vi "Test.vi"() -> ()   [LabVIEW 2013, in "Standard Editor.lvlib" / "splash screen.lvlib"]
uses:
  splash screen.lvlib
  notifier data.ctl
panel:
  out "error out":errorcluster
  in  "error in":errorcluster
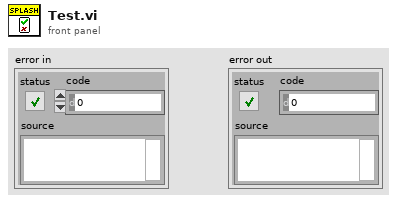
[diagram p1: front panel]
types:
  T1 = typedef "Standard Editor.lvlib/splash screen.lvlib/splash screen.ctl" = cluster{"reference":refnum<vi>, "update notifier":refnum<notifier>, "Initialized":bool}
  T2 = typedef "Standard Editor.lvlib/splash screen.lvlib/notifier data.ctl" = cluster{"Text":string, "percent":dbl}
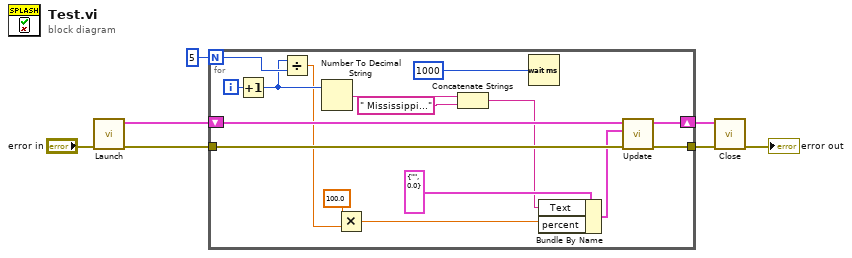
[diagram p0: block diagram]
diagram:
  n1 = call "Launch.vi"("error in"="error in") -> ("error out"=w5:errorcluster, "SplashScreen"=w6:T1)  [unwired: 9 in]
  n2 = for {
    N: 5 -> [w20]
    tunnel: w5 -> [w22]
    tunnel: [w15] -> w2
    shift-right: [w16] -> w3
    shift-left: w6 -> [w23]
    i -> [w21]
    n3 = Increment(x=w21) -> (x+1=w19:i32)
    n4 = Divide(x=w19, y=w20) -> (x/y=w10:dbl)
    n5 = Number To Decimal String(number=w19) -> (decimal integer string=w12:string)  [unwired: 1 in]
    n6 = Multiply(x=100.0, y=w10) -> (x*y=w8:dbl)
    n7 = Concatenate Strings(w12, " Mississippi...") -> (w11:string)
    n8 = Wait (ms)(milliseconds to wait=u32 1000) -> ()  [unwired: 1 out]
    n9 = Bundle By Name(cluster=T2 {"Text"="", "percent"=0.0} ("Update"), "Text"=w11, "percent"=w8) -> (w17:T2)
    n10 = call "Update.vi"("error in"=w22, "Update"=w17, "SplashScreen in"=w23) -> ("error out"=w15:errorcluster, "SplashScreen out"=w16:T1)  [unwired: 7 in]
  }
  n11 = call "Close.vi"("error in"=w2, "SplashScreen"=w3) -> ("error out"=→"error out":errorcluster)  [unwired: 8 in, 1 out]
